vi "TurretCoordinateTransform.vi"(2 "robot heading [0,360]":dbl, 3 "turret heading [0, 360]":dbl) -> (0 "Ly":dbl, 1 "Lx":dbl)   [LabVIEW 2019]
panel:
  in  "radius":dbl
  in  "ty'":dbl
  in  "tx'":dbl
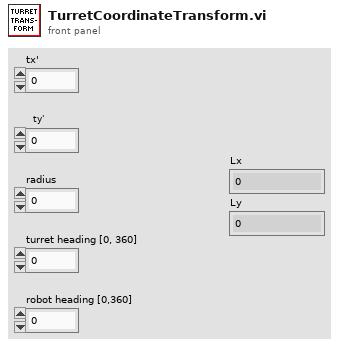
[diagram p1: front panel]
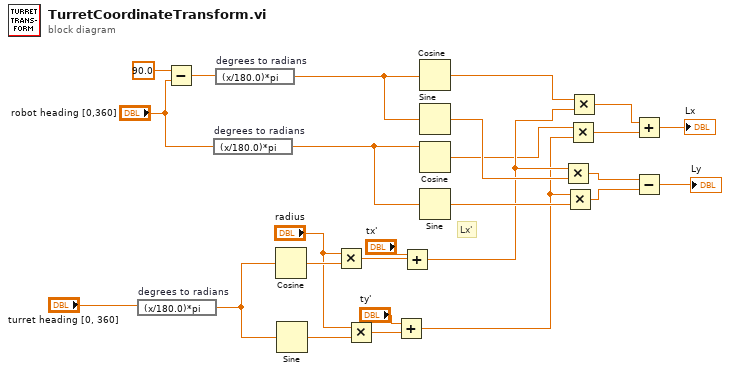
[diagram p0: block diagram]
diagram:
  # "Lx'"
  n1 = expression code="(x/180.0)*pi" "degrees to radians"("turret heading [0, 360]") -> (w22:dbl)
  n2 = Subtract(x=90.0, y="robot heading [0,360]") -> (x-y=w16:dbl)
  n3 = expression code="(x/180.0)*pi" "degrees to radians"("robot heading [0,360]") -> (w10:dbl)
  n4 = expression code="(x/180.0)*pi" "degrees to radians"(w16) -> (w15:dbl)
  n5 = Cosine(x=w22) -> (cos(x)=w25:dbl)
  n6 = Sine(x=w22) -> (sin(x)=w20:dbl)
  n7 = Multiply(x="radius", y=w25) -> (x*y=w23:dbl)
  n8 = Multiply(x="radius", y=w20) -> (x*y=w19:dbl)
  n9 = Add(x="ty'", y=w19) -> (x+y=w1:dbl)
  n10 = Add(x="tx'", y=w23) -> (x+y=w3:dbl)
  n11 = Cosine(x=w15) -> (cos(x)=w4:dbl)
  n12 = Sine(x=w15) -> (sin(x)=w12:dbl)
  n13 = Cosine(x=w10) -> (cos(x)=w2:dbl)
  n14 = Sine(x=w10) -> (sin(x)=w9:dbl)
  n15 = Multiply(x=w3, y=w12) -> (x*y=w11:dbl)
  n16 = Multiply(x=w1, y=w9) -> (x*y=w8:dbl)
  n17 = Multiply(x=w2, y=w1) -> (x*y=w6:dbl)
  n18 = Multiply(x=w4, y=w3) -> (x*y=w5:dbl)
  n19 = Add(x=w5, y=w6) -> (x+y=→"Lx":dbl)
  n20 = Subtract(x=w11, y=w8) -> (x-y=→"Ly":dbl)
